vi "AlternatingLEDs.vi"() -> ()   [LabVIEW 2014]
panel:
  in  "Number of milliseconds between switching":dbl(slide) scale=0.0..100.0
  in  "stop":bool
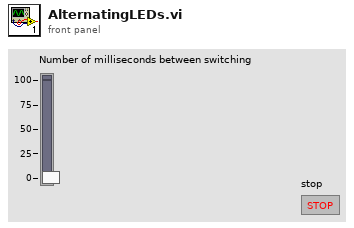
[diagram p1: front panel]
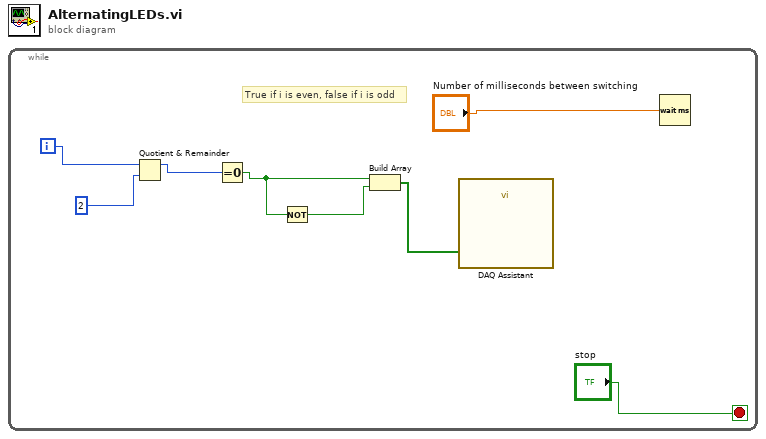
[diagram p0: block diagram]
diagram:
  n1 = while {
    i -> [w8]
    stop <- "stop" stop-if-true
    # "True if i is even, false if i is odd"
    n2 = Quotient & Remainder(x=w8, y=2) -> (x-y*floor(x/y)=w6:i32)  [unwired: 1 out]
    n3 = Equal To 0?(x=w6) -> (x = 0?=w3:bool)
    n4 = Not(x=w3) -> (.not. x?=w2:bool)
    n5 = Build Array(w3, w2) -> (w5:bool[])
    n6 = call "DAQ Assistant"("data"=w5) -> ()  [unwired: 17 in, 2 out]
    n7 = Wait (ms)(milliseconds to wait="Number of milliseconds between switching") -> ()  [unwired: 1 out]
  }
